vi "Request Summary.vi"(8 "error in (no error)":errorcluster, 10 "Promise":refnum<class "Promise.lvclass">, 11 "VMR Actor in":refnum<class "VMR Actor.lvclass">) -> (0 "error out":errorcluster, 3 "VMR Actor out":refnum<class "VMR Actor.lvclass">)   [LabVIEW 2022 SP3, in "VMR Server.lvlib" / "VMR Actor.lvclass"]
uses:
  VMR Actor.lvclass
  <vilib>/IlluminatedG/IG Promises/Promises/Promise/Promise.lvclass
  <vilib>/IlluminatedG/IG VoicemeeterRemote API/VoiceMeeterRemote/Direction.ctl
  VMR Actor.lvclass/VMR Actor.ctl
  VMR Server Shared/Channel.ctl
  AudioSummaryValue/AudioSummaryValue.lvclass
  C:/Program Files (x86)/National Instruments/LabVIEW 2022/vi.lib/IlluminatedG/IG Promises/Promises/Value/Value.lvclass
  <vilib>/IlluminatedG/IG VoicemeeterRemote API/VoiceMeeterRemote/VoiceMeeterRemote/VoiceMeeterRemote.lvclass
  <vilib>/IlluminatedG/IG VoicemeeterRemote API/VoiceMeeterRemote/VoiceMeeterRemote.lvlib
  VMR Server Shared/VMR Server Shared.lvlib
  C:/dev/lv/2022/touchcontrol/VMR Server/AudioSummaryValue/AudioSummaryValue.lvclass
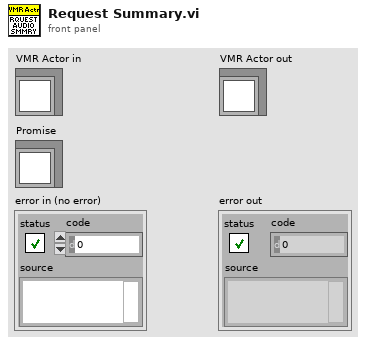
[diagram p1: front panel]
types:
  T1 = typedef "VoiceMeeterRemote.lvlib/Direction.ctl" = enum16{"Input", "Output"}
  T2 = typedef "VoiceMeeterRemote.lvlib/Levels.ctl" = cluster{"Input Pre Fader":T3[], "Input Post Fader":T3[], "Input Post Mute":T3[], "Output":T3[]}
  T3 = typedef "VoiceMeeterRemote.lvlib/Device Channels.ctl" = cluster{"Values":sgl[]}
  T4 = typedef "VMR Server Shared.lvlib/Channel.ctl" = cluster{"Gain":dbl, "Muted":bool, "Levels":cluster{"L":dbl, "R":dbl}}
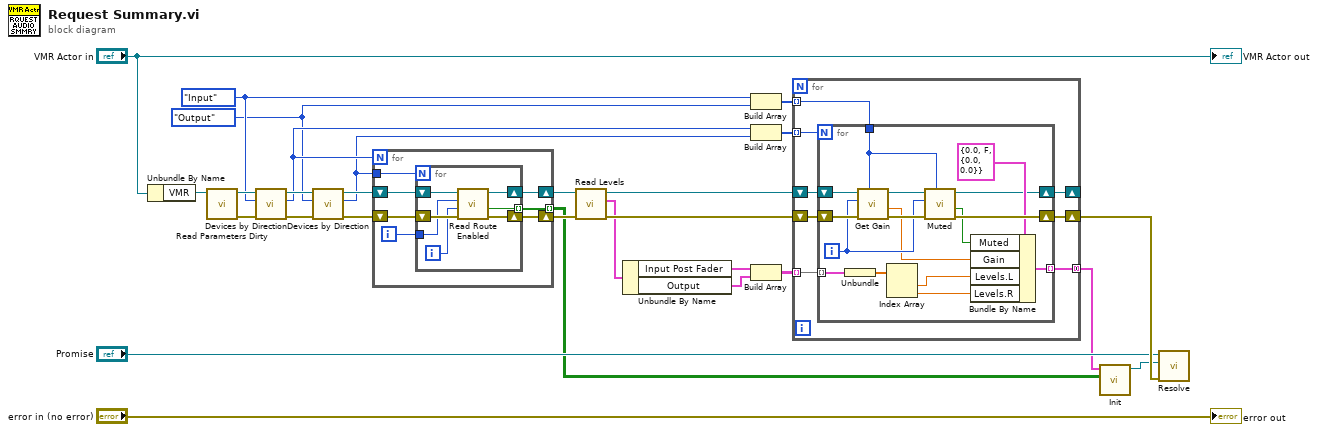
[diagram p0: block diagram]
diagram:
  w12 = Direction."Output" ("Direction")
  w13 = Direction."Input" ("Direction")
  n1 = Unbundle By Name("VMR Actor in") -> ("VMR"=w23:refnum<class "VoiceMeeterRemote.lvclass">)
  n2 = call <vilib>:"Read Parameters Dirty.vi"("VoiceMeeterRemote in"=w23) -> ("error out"=w10:errorcluster, "VoiceMeeterRemote out"=w22:refnum<class "VoiceMeeterRemote.lvclass">)  [unwired: 8 in, 1 out]
  n3 = call <vilib>:"Devices by Direction.vi"("error in (no error)"=w10, "Direction"=w13, "VoiceMeeterRemote in"=w22) -> ("error out"=w9:errorcluster, "Device Count"=w16:i32, "VoiceMeeterRemote out"=w21:refnum<class "VoiceMeeterRemote.lvclass">)  [unwired: 6 in]
  n4 = call <vilib>:"Devices by Direction.vi"("error in (no error)"=w9, "Direction"=w12, "VoiceMeeterRemote in"=w21) -> ("error out"=w8:errorcluster, "Device Count"=w15:i32, "VoiceMeeterRemote out"=w20:refnum<class "VoiceMeeterRemote.lvclass">)  [unwired: 6 in]
  n5 = for {
    N: w16 -> [_]
    shift-right: [w32] -> w19
    shift-left: w20 -> [w34]
    tunnel: w15 -> [w35]
    tunnel: [w31] -> w4 mode=indexing
    shift-right: [w29] -> w7
    shift-left: w8 -> [w30]
    i -> [w33]
    n6 = for {
      N: w35 -> [_]
      shift-right: [w38] -> w32
      shift-left: w34 -> [w41]
      tunnel: w33 -> [w40]
      tunnel: [w37] -> w31 mode=indexing
      shift-right: [w36] -> w29
      shift-left: w30 -> [w42]
      i -> [w39]
      n7 = call <vilib>:"Read Route Enabled.vi"("error in (no error)"=w42, "Output Index"=w39, "Input Index"=w40, "VoiceMeeterRemote in"=w41) -> ("error out"=w36:errorcluster, "Route Enabled?"=w37:bool, "VoiceMeeterRemote out"=w38:refnum<class "VoiceMeeterRemote.lvclass">)  [unwired: 4 in, 1 out]
    }
  }
  n8 = call <vilib>:"Read Levels.vi"("error in (no error)"=w7, "VoiceMeeterRemote in"=w19) -> ("error out"=w28:errorcluster, "Levels"=w17:T2, "VoiceMeeterRemote out"=w18:refnum<class "VoiceMeeterRemote.lvclass">)  [unwired: 7 in]
  n9 = Unbundle By Name(w17) -> ("Input Post Fader"=w2:T3[], "Output"=w1:T3[])
  n10 = Build Array(w13, w12) -> (w11:T1[])
  n11 = Build Array(w16, w15) -> (w14:i32[])
  n12 = Build Array(w2, w1) -> (w3:T3[][])
  n13 = for {
    tunnel: w14 -> [w49] mode=indexing
    tunnel: w3 -> [w48] mode=indexing
    tunnel: w11 -> [w47] mode=indexing
    tunnel: [w46] -> w5 mode=concatenating
    shift-right: [w45] -> _
    shift-left: w18 -> [w50]
    shift-right: [w43] -> w27
    shift-left: w28 -> [w44]
    n14 = for {
      N: w49 -> [_]
      shift-right: [w51] -> w45
      shift-left: w50 -> [w63]
      tunnel: w48 -> [w62] mode=indexing
      tunnel: w47 -> [w56]
      tunnel: [w52] -> w46 mode=indexing
      shift-right: [w66] -> w43
      shift-left: w44 -> [w64]
      i -> [w55]
      n15 = Unbundle(w62) -> ("Values"=w61:sgl[])
      n16 = call <vilib>:"Get Gain.vi"("Direction"=w56, "error in (no error)"=w64, "Index"=w55, "VoiceMeeterRemote in"=w63) -> ("error out"=w65:errorcluster, "Value"=w54:sgl, "VoiceMeeterRemote out"=w59:refnum<class "VoiceMeeterRemote.lvclass">)  [unwired: 5 in]
      n17 = Index Array(array=w61) -> (element #1=w53:sgl, element #2=w58:sgl)  [unwired: 2 in]
      n18 = call <vilib>:"Muted.vi"("Direction"=w56, "error in (no error)"=w65, "Index"=w55, "VoiceMeeterRemote in"=w59) -> ("error out"=w66:errorcluster, "Muted?"=w57:bool, "VoiceMeeterRemote out"=w51:refnum<class "VoiceMeeterRemote.lvclass">)  [unwired: 5 in]
      n19 = Bundle By Name(cluster=T4 {"Gain"=0.0, "Muted"=FALSE, "Levels"={"L"=0.0, "R"=0.0}} ("Channel"), "Muted"=w57, "Gain"=w54, "Levels.L"=w53, "Levels.R"=w58) -> (w52:T4)
    }
  }
  n20 = call "Init.vi"("Route"=w4, "Channels"=w5) -> ("AudioSummaryValue out"=w25:refnum<class "AudioSummaryValue.lvclass">)  [unwired: 8 in, 1 out]
  n21 = call <vilib>:"Resolve.vi"("error in (no error)"=w27, "Result"=w25, "Promise in"="Promise") -> ()  [unwired: 7 in, 2 out]
  "error out" <- "error in (no error)"
  "VMR Actor out" <- "VMR Actor in"
